vi "labview-01-sample.vi"() -> ()   [LabVIEW 2020]
panel:
  out "Output-Subtract":dbl
  out "Output-Add":dbl
  in  "Input-B":dbl
  in  "Input-A":dbl
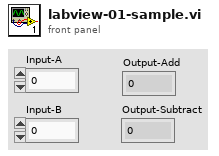
[diagram p1: front panel]
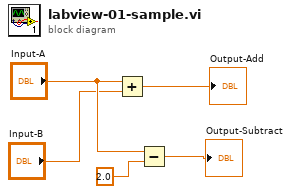
[diagram p0: block diagram]
diagram:
  n1 = Add(x="Input-A", y="Input-B") -> (x+y=→"Output-Add":dbl)
  n2 = Subtract(x="Input-A", y=2.0) -> (x-y=→"Output-Subtract":dbl)
